vi "Disabled.vi"(7 "Robot Mode":T2, 10 "Match Info":T1={"Autonomous Elapsed Seconds"=0.0, "TeleOp Elapsed Seconds"=0.0, "Disabled Elapsed Seconds"=0.0, "Visited Autonomous"=FALSE, "Visited TeleOp"=FALSE, "Visited Disabled"=FALSE, "Autonomous Settings"={"Autonomous Style"=enum."Independent", "VI Refnum"=refnum}}, 11 "Call Context":T3) -> ()   [LabVIEW 2011]
doc: "This VI is called each time a disabled packet is received from the DS. It is often used to prepare for the next robot mode, to calibrate sensors, etc."
uses:
  <vilib>/Rock Robotics/WPI/DriverStation/WPI_DriverStationDerivedRobotMode.ctl
  <vilib>/Rock Robotics/WPI/DriverStation/WPI_DriverStationRobotMode.ctl
  <vilib>/Rock Robotics/WPI/DriverStation/WPI_DriverStationMatch Info.ctl
  Robot Global Data.vi
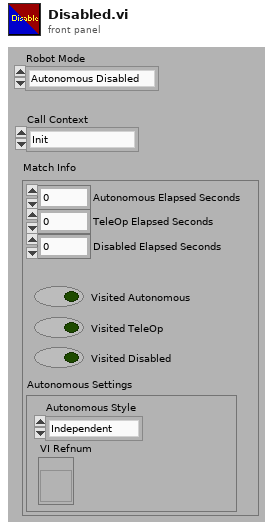
[diagram p1: front panel]
types:
  T1 = typedef "WPI_DriverStationMatch Info.ctl" = cluster{"Autonomous Elapsed Seconds":dbl, "TeleOp Elapsed Seconds":dbl, "Disabled Elapsed Seconds":dbl, "Visited Autonomous":bool, "Visited TeleOp":bool, "Visited Disabled":bool, "Autonomous Settings":cluster{"Autonomous Style":enum16{"Iterative", "Independent"}, "VI Refnum":refnum<vi>}}
  T2 = typedef "WPI_DriverStationRobotMode.ctl" = enum16{"Autonomous Disabled", "Autonomous Enabled", "Teleop Disabled", "Teleop Enabled", "Timeout", "Finish"}
  T3 = typedef "WPI_DriverStationDerivedRobotMode.ctl" = enum16{"Init", "Execute", "Stop"}
  T4 = typedef "WPI_MotorControlDeviceRef.ctl" = cluster{"DeviceStatus":errorcluster, "Type":enum16{"PWM", "CAN"}, "PWM":cluster{"Digital Module":T5, "PWM Channel":T6, "DeadBand":T7}, "CAN":cluster{"Device Number":u8, "Control Mode":T8, "Semaphore":T9, "Max Vout":dbl}, "Invert":bool, "TransformRef":T10, "InvTransformRef":T10}
  T5 = typedef "FPGA_TypedefDigitalModule.ctl" = enum16{"Digital Module 1", "Digital Module 2"}
  T6 = typedef "FPGA_DIOPWMChannel.ctl" = enum8{"PWM 1", "PWM 2", "PWM 3", "PWM 4", "PWM 5", "PWM 6", "PWM 7", "PWM 8", "PWM 9", "PWM 10", "Invalid"}
  T7 = typedef "WPI_PWMDeadband.ctl" = cluster{"Name":string, "maxPositivePwm":i32, "minPositivePwm":i32, "centerPwm":i32, "maxNegativePwm":i32, "minNegativePwm":i32, "angularRange":u16}
  T8 = typedef "WPI_CANJaguar_ControlMode.ctl" = enum8{"Percent VBus", "Current", "Speed", "Position", "Voltage"}
  T9 = typedef "Semaphore RefNum" = refnum<k1>
  T10 = typedef "WPI_PWMTransform_ConPane.ctl" = refnum<vi>
  T11 = typedef "WPI_JoystickDevRef.ctl" = cluster{"Device":T12}
  T12 = typedef "WPI_JoystickDeviceEnum.ctl" = enum16{"USB 1", "USB 2", "USB 3", "USB 4", "Kinect 1", "Kinect 2"}
  T13 = typedef "WPI_JoystickButtonState.ctl" = cluster{"Button 1":bool, "Button 2":bool, "Button 3":bool, "Button 4":bool, "Button 5":bool, "Button 6":bool, "Button 7":bool, "Button 8":bool, "Button 9":bool, "Button 10":bool, "Button 11":bool, "Button 12":bool}
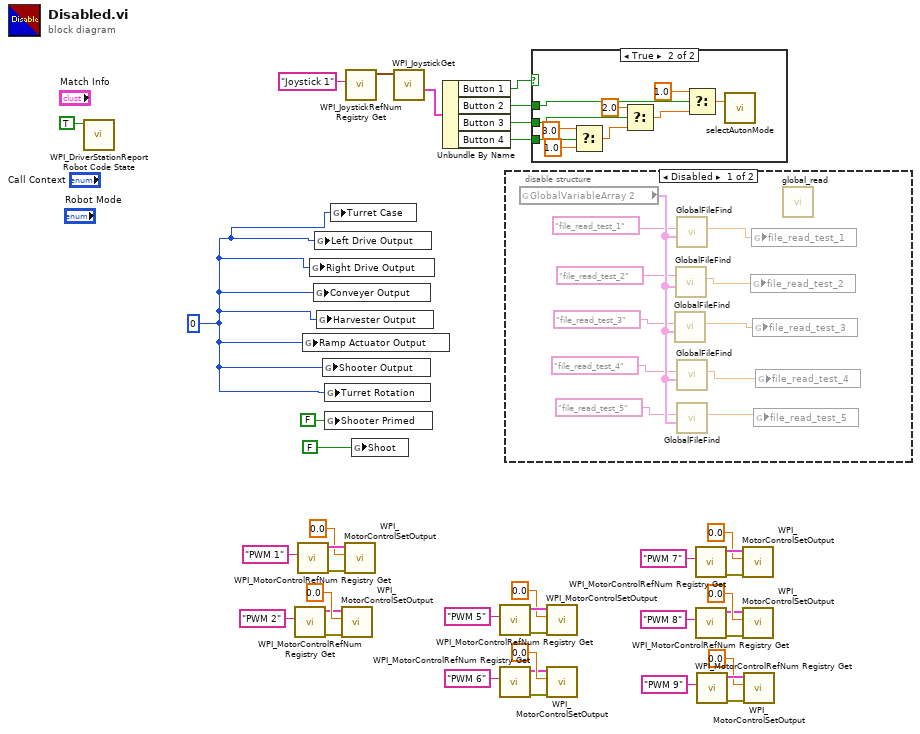
[diagram p0: block diagram]
diagram:
  w8 = 0
  n1 = call <vilib>:"WPI_DriverStationReport Robot Code State.vi"("Disabled"=TRUE ("Autonomous")) -> ()  [unwired: 10 in, 1 out]
  n2 = call <vilib>:"WPI_MotorControlRefNum Registry Get.vi"("refnum name"="PWM 2") -> ("error out"=w32:errorcluster, "MotorControlDevRef"=w31:T4)  [unwired: 9 in]
  n3 = call <vilib>:"WPI_MotorControlRefNum Registry Get.vi"("refnum name"="PWM 1") -> ("error out"=w37:errorcluster, "MotorControlDevRef"=w38:T4)  [unwired: 9 in]
  n4 = global write "Robot Global Data.vi" "Ramp Actuator Output"(w8) -> ()
  n5 = global write "Robot Global Data.vi" "Right Drive Output"(w8) -> ()
  n6 = global write "Robot Global Data.vi" "Conveyer Output"(w8) -> ()
  n7 = global write "Robot Global Data.vi" "Left Drive Output"(w8) -> ()
  n8 = global write "Robot Global Data.vi" "Harvester Output"(w8) -> ()
  n9 = global write "Robot Global Data.vi" "Shooter Output"(w8) -> ()
  n10 = global write "Robot Global Data.vi" "Turret Rotation"(w8) -> ()
  n11 = global write "Robot Global Data.vi" "Shooter Primed"(FALSE ("Shooter Primed")) -> ()
  n12 = global write "Robot Global Data.vi" "Turret Case"(w8) -> ()
  n13 = call <vilib>:"WPI_MotorControlSetOutput.vi"("error in (no error)"=w32, "Output"=0.0, "MotorControlDevRef"=w31) -> ()  [unwired: 7 in, 2 out]
  n14 = call <vilib>:"WPI_MotorControlSetOutput.vi"("error in (no error)"=w37, "Output"=0.0, "MotorControlDevRef"=w38) -> ()  [unwired: 7 in, 2 out]
  n15 = call <vilib>:"WPI_JoystickRefNum Registry Get.vi"("refnum name"="Joystick 1") -> ("JoystickDevRef"=w6:T11)  [unwired: 9 in, 1 out]
  n16 = global write "Robot Global Data.vi" "Shoot"(FALSE ("Shooter Primed")) -> ()
  n17 = call <vilib>:"WPI_JoystickGet.vi"("JoystickDevRef"=w6) -> ("Buttons"=w5:T13)  [unwired: 4 in, 2 out]
  n18 = Unbundle By Name(w5) -> ("Button 1"=w4:bool, "Button 2"=w3:bool, "Button 3"=w2:bool, "Button 4"=w1:bool)
  n19 = call <vilib>:"WPI_MotorControlRefNum Registry Get.vi"("refnum name"="PWM 5") -> ("error out"=w29:errorcluster, "MotorControlDevRef"=w30:T4)  [unwired: 9 in]
  n20 = call <vilib>:"WPI_MotorControlRefNum Registry Get.vi"("refnum name"="PWM 6") -> ("error out"=w24:errorcluster, "MotorControlDevRef"=w23:T4)  [unwired: 9 in]
  n21 = disable-structure shown="Disabled" {
    frame Disabled {
      n22 = global read "Robot Global Data.vi" "GlobalVariableArray 2"() -> (w50:cluster{"name":string, "va;":dbl}[])
      n23 = call "GlobalFileFind.vi"("GlobalVariableArray 2"=w50, "VariableNameLookup"="file_read_test_3") -> ("VariableValueOut"=w41:dbl)  [unwired: 9 in]
      n24 = call "GlobalFileFind.vi"("GlobalVariableArray 2"=w50, "VariableNameLookup"="file_read_test_2") -> ("VariableValueOut"=w40:dbl)  [unwired: 9 in]
      n25 = call "GlobalFileFind.vi"("GlobalVariableArray 2"=w50, "VariableNameLookup"="file_read_test_1") -> ("VariableValueOut"=w44:dbl)  [unwired: 9 in]
      n26 = call "GlobalFileFind.vi"("GlobalVariableArray 2"=w50, "VariableNameLookup"="file_read_test_4") -> ("VariableValueOut"=w42:dbl)  [unwired: 9 in]
      n27 = call "GlobalFileFind.vi"("GlobalVariableArray 2"=w50, "VariableNameLookup"="file_read_test_5") -> ("VariableValueOut"=w43:dbl)  [unwired: 9 in]
      n28 = global write "Robot Global Data.vi" "file_read_test_2"(w40) -> ()
      n29 = global write "Robot Global Data.vi" "file_read_test_1"(w44) -> ()
      n30 = global write "Robot Global Data.vi" "file_read_test_3"(w41) -> ()
      n31 = global write "Robot Global Data.vi" "file_read_test_5"(w43) -> ()
      n32 = global write "Robot Global Data.vi" "file_read_test_4"(w42) -> ()
      n33 = call "global_read.vi"() -> ()  [unwired: 12 in]
    }
    frame Enabled {
    }
  }
  n34 = case shown="True" w4 {
    tunnel: w3 -> [_ w57]
    tunnel: w2 -> [_ w55]
    tunnel: w1 -> [_ w60]
    frame False {
    }
    frame True {
      n35 = Select(t=3.0, s=w60, f=1.0) -> (s? t:f=w53:dbl)
      n36 = Select(t=2.0, s=w55, f=w53) -> (s? t:f=w52:dbl)
      n37 = Select(t=1.0, s=w57, f=w52) -> (s? t:f=w51:dbl)
      n38 = call "selectAutonMode.vi"("Auton File"=w51) -> ()  [unwired: 2 in]
    }
  }
  n39 = call <vilib>:"WPI_MotorControlSetOutput.vi"("error in (no error)"=w29, "Output"=0.0, "MotorControlDevRef"=w30) -> ()  [unwired: 7 in, 2 out]
  n40 = call <vilib>:"WPI_MotorControlSetOutput.vi"("error in (no error)"=w24, "Output"=0.0, "MotorControlDevRef"=w23) -> ()  [unwired: 7 in, 2 out]
  n41 = call <vilib>:"WPI_MotorControlRefNum Registry Get.vi"("refnum name"="PWM 7") -> ("error out"=w21:errorcluster, "MotorControlDevRef"=w22:T4)  [unwired: 9 in]
  n42 = call <vilib>:"WPI_MotorControlRefNum Registry Get.vi"("refnum name"="PWM 8") -> ("error out"=w16:errorcluster, "MotorControlDevRef"=w15:T4)  [unwired: 9 in]
  n43 = call <vilib>:"WPI_MotorControlRefNum Registry Get.vi"("refnum name"="PWM 9") -> ("error out"=w13:errorcluster, "MotorControlDevRef"=w14:T4)  [unwired: 9 in]
  n44 = call <vilib>:"WPI_MotorControlSetOutput.vi"("error in (no error)"=w21, "Output"=0.0, "MotorControlDevRef"=w22) -> ()  [unwired: 7 in, 2 out]
  n45 = call <vilib>:"WPI_MotorControlSetOutput.vi"("error in (no error)"=w16, "Output"=0.0, "MotorControlDevRef"=w15) -> ()  [unwired: 7 in, 2 out]
  n46 = call <vilib>:"WPI_MotorControlSetOutput.vi"("error in (no error)"=w13, "Output"=0.0, "MotorControlDevRef"=w14) -> ()  [unwired: 7 in, 2 out]
